vi "Library Log Error to Window.vi"(11 "error in (no error)":errorcluster) -> (4 "error?":bool, 15 "dup error":errorcluster)   [LabVIEW 2012]
doc: "Logs the provided error to a log window if the error is set. The logged error message will be prefixed with the current time."
uses:
  glb_Library Configuration Globals.vi
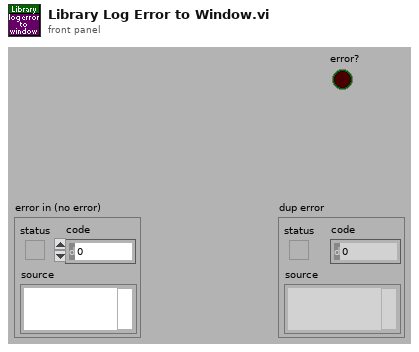
[diagram p1: front panel]
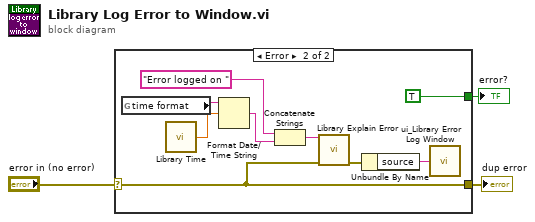
[diagram p0: block diagram]
diagram:
  n1 = case shown="Error" "error in (no error)" {
    selector: "error in (no error)" -> [w4 w7]
    tunnel: [_ TRUE ("error?")] -> w2
    tunnel: [w4 w7] -> w1
    frame No Error {
    }
    frame Error {
      n2 = global read "glb_Library Configuration Globals.vi" "time format"() -> (w10:string)
      n3 = call "Library Time.vi"() -> ("time"=w11:dbl)  [unwired: 1 in]
      n4 = Format Date/Time String(time format string (%c)=w10, seconds (now)=w11) -> (date/time string=w12:string)  [unwired: 1 in]
      n5 = Concatenate Strings("Error logged on " ("time format string (%c)"), w12) -> (w8:string)
      n6 = call "Library Explain Error.vi"("explanation prefix (none)"=w8, "error in (no error)"=w7) -> ("explained error"=w6:errorcluster)  [unwired: 13 in]
      n7 = Unbundle By Name(w6) -> ("source"=w5:string)
      n8 = call "ui_Library Error Log Window.vi"("error message"=w5) -> ()  [unwired: 1 in]
    }
  }
  "error?" <- w2
  "dup error" <- w1
